vi "Init.vi"(8 "error in (no error)":errorcluster caption="entrée d'erreur (pas d'erreur)", 11 "Class Spectrum_Analyser RS306B en entrée":refnum<class "Class Spectrum_Analyser RS306B.lvclass">) -> (0 "error out":errorcluster caption="sortie d'erreur", 3 "Class Spectrum_Analyser RS306B en sortie":refnum<class "Class Spectrum_Analyser RS306B.lvclass">)   [LabVIEW 2020, in "Library Instrument & Equipement.lvlib" / "Library Spectrum Analyser.lvlib" / "Class Spectrum_Analyser RS306B.lvclass"]
uses:
  Class Spectrum_Analyser RS306B.lvclass
  C:/Users/ngarcin/OneDrive - Altyor/Standard TB/Class/Spectrum Analyser/Class Spectrum Analyser (Default)/Class Spectrum Analyser (Default).lvclass
  Class Spectrum_Analyser RS306B.lvclass/Class Spectrum_Analyser RS306B.ctl
  Library Spectrum Analyser.lvlib
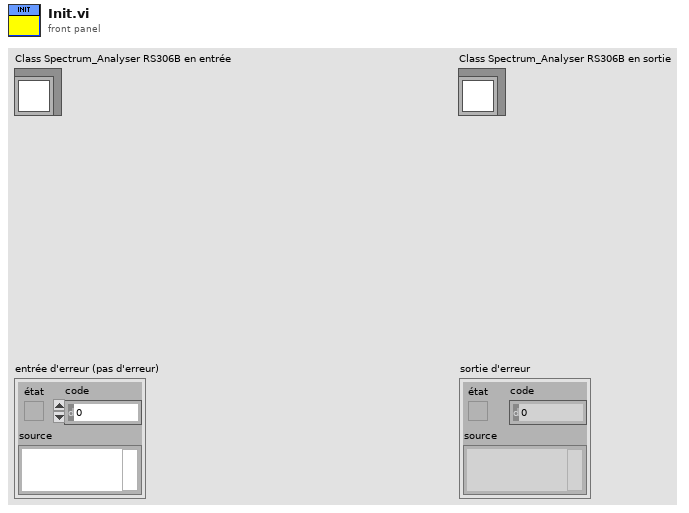
[diagram p1: front panel]
types:
  T1 = enum16{"SEARCH ON", "SEARCH OFF", "SEARCH TRACE", "SEARCH CRITERIA", "SEARCH THRESHOLD", "BEEP ON MATCH ON", "BEEP ON MATCH OFF", "STOP ON MATCH ON", "STOP ON MATCH OFF", "AUTOSAVE ACQ DATA ON MATCH ON", "AUTOSAVE ACQ DATA ON MATCH OFF", "AUTOSAVE TRACE ON MATCH ON", "AUTOSAVE TRACE ON MATCH OFF", "AUTOSAVE PICTURE ON MATCH ON", "AUTOSAVE PICTURE ON MATCH OFF", "SAVE SEARCH MASK TO FILE (SET)", "LOAD SEARCH MASK FROM FILE (SET)", "SEARCH RESULTS (READ)"}
  T2 = enum16{"<  THRESHOLD", "> THRESHOLD", "INSIDE MASK", "OUTSIDE MASK"}
  T3 = enum16{"NORMAL", "AVERAGE", "MAX HOLD", "MIN HOLD", "AVERAGE LOG"}
  T4 = enum16{"TRACE FUNCTION", "TRACE DETECTION", "SELECT TRACE", "TRACE ON", "TRACE OFF", "FREEZE ON", "FREEZE OFF", "AVERAGE COUNT", "CLEAR AVE/MAX/MIN (SET)", "CLEAR TRACES (SET)", "LEFT OPERAND", "RIGHT OPERAND"}
  T5 = enum16{"+PEAK", "-PEAK", "AVERAGE", "SAMPLE", "CISPR AVG", "CISPR PK", "CISPR QPK", "AVERAGE LOG"}
  T6 = enum16{"REFERENCE LEVEL", "RF ATTENUATION", "AUTO ATTENUATION ON", "AUTO ATTENUATION OFF", "PREAMP ON", "PREAMP OFF", "VERTICAL UNITS"}
  T7 = enum16{"CENTER FREQUENCY", "FREQUENCY SPAN", "RESOLUTION BW", "MAX REAL TIME SPAN (SET)", "START FREQUENCY", "STOP FREQUENCY", "FREQ STEP SIZE", "AUTO FREQ STEP ON", "AUTO FREQ STEP OFF", "AUTO RES BW ON", "AUTO RES BW OFF", "FFT WINDOW TYPE", "# POINTS", "RBW PROCESS ON", "RBW PROCESS OFF", "GAIN/BW OPTIMIZATION"}
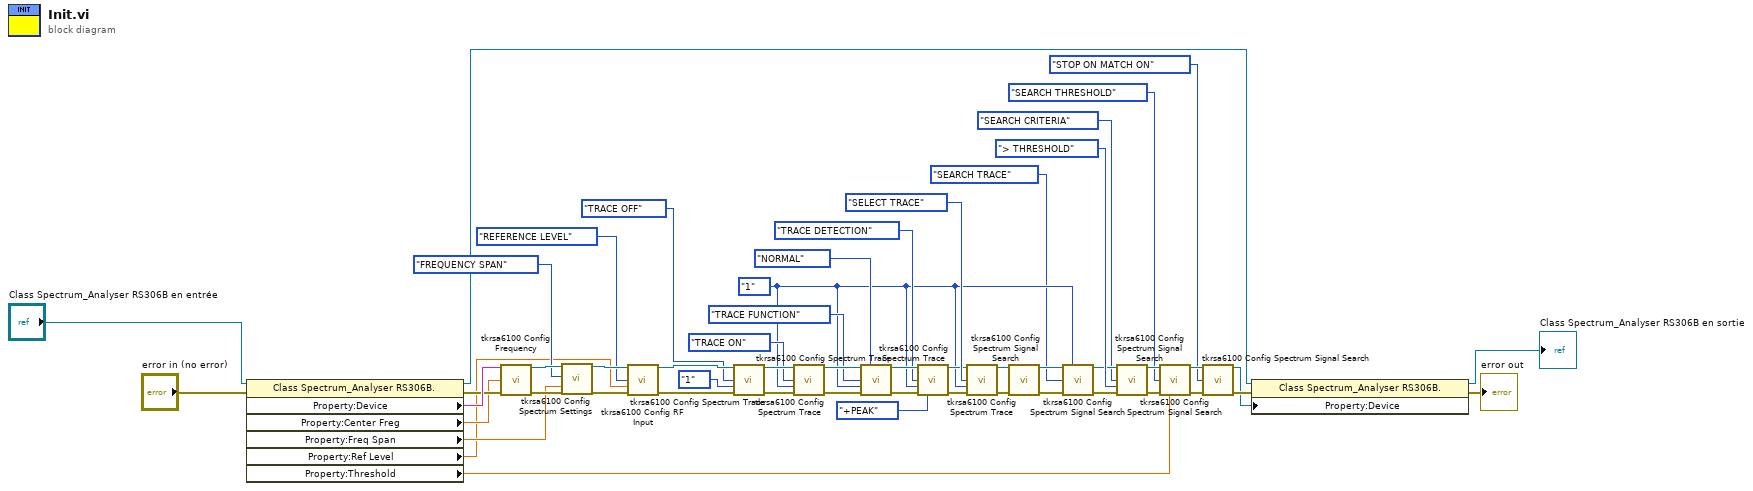
[diagram p0: block diagram]
diagram:
  w27 = enum16{"1", "2", "3", "MATH", "SGRAM"}."1" ("Trace # (1)")
  n1 = property class="Class Spectrum_Analyser RS306B."(reference="Class Spectrum_Analyser RS306B en entrée", error in="error in (no error)") -> (reference out=w8:refnum<class "Class Spectrum_Analyser RS306B.lvclass">, error out=w11:errorcluster, "Property:Device"=w12:string, "Property:Center Freg"=w4:dbl, "Property:Freq Span"=w3:dbl, "Property:Ref Level"=w2:dbl, "Property:Threshold"=w1:dbl)
  n2 = call "tkrsa6100 Config Frequency.vi"("VISA Resource Name"=w12, "Msmt Freq (MHz)\n(1000)"=w4, "error in (no error)"=w11) -> ("dup VISA Resource Name"=w53:refnum<visa-resource-name>, "error out"=w52:errorcluster)  [unwired: 10 in, 1 out]
  n3 = call "tkrsa6100 Config Spectrum Settings.vi"("VISA Resource Name"=w53, "Spectrum Settings\n (CENTER FREQUENCY)"=T7."FREQUENCY SPAN" ("Spectrum Settings\n (CENTER FREQUENCY)"), "Freq Span\n(MHz)(40)"=w3, "error in (no error)"=w52) -> ("dup VISA Resource Name"=w51:refnum<visa-resource-name>, "error out"=w50:errorcluster)  [unwired: 13 in, 1 out]
  n4 = call "tkrsa6100 Config RF Input.vi"("VISA Resource Name"=w51, "Input Settings\n(REFERENCE LEVEL)"=T6."REFERENCE LEVEL" ("Input Settings\n(REFERENCE LEVEL)"), "Ref Level (0)"=w2, "error in (no error)"=w50) -> ("dup VISA Resource Name"=w49:refnum<visa-resource-name>, "error out"=w48:errorcluster)  [unwired: 9 in, 1 out]
  n5 = call "tkrsa6100 Config Spectrum Trace.vi"("VISA Resource Name"=w49, "Trace Setting\n(TRACE FUNCTION)"=T4."TRACE OFF" ("Trace Setting\n(TRACE FUNCTION)"), "Trace # (1)"=enum16{"1", "2", "3", "MATH", "SGRAM"}."1", "error in (no error)"=w48) -> ("dup VISA Resource Name"=w43:refnum<visa-resource-name>, "error out"=w42:errorcluster)  [unwired: 9 in, 1 out]
  n6 = call "tkrsa6100 Config Spectrum Trace.vi"("VISA Resource Name"=w43, "Trace Setting\n(TRACE FUNCTION)"=T4."TRACE ON" ("Trace Setting\n(TRACE FUNCTION)"), "Trace # (1)"=w27, "error in (no error)"=w42) -> ("dup VISA Resource Name"=w38:refnum<visa-resource-name>, "error out"=w39:errorcluster)  [unwired: 9 in, 1 out]
  n7 = call "tkrsa6100 Config Spectrum Trace.vi"("VISA Resource Name"=w38, "Trace Function\n(NORMAL)"=T3."NORMAL" ("Trace Function\n(NORMAL)"), "Trace Setting\n(TRACE FUNCTION)"=T4."TRACE FUNCTION" ("Trace Setting\n(TRACE FUNCTION)"), "Trace # (1)"=w27, "error in (no error)"=w39) -> ("dup VISA Resource Name"=w34:refnum<visa-resource-name>, "error out"=w36:errorcluster)  [unwired: 8 in, 1 out]
  n8 = call "tkrsa6100 Config Spectrum Trace.vi"("VISA Resource Name"=w34, "Trace Setting\n(TRACE FUNCTION)"=T4."TRACE DETECTION" ("Trace Setting\n(TRACE FUNCTION)"), "Trace # (1)"=w27, "error in (no error)"=w36, "Trace Detection\n(+PEAK)"=T5."+PEAK" ("Trace Detection\n(+PEAK)")) -> ("dup VISA Resource Name"=w33:refnum<visa-resource-name>, "error out"=w35:errorcluster)  [unwired: 8 in, 1 out]
  n9 = call "tkrsa6100 Config Spectrum Trace.vi"("VISA Resource Name"=w33, "Trace Setting\n(TRACE FUNCTION)"=T4."SELECT TRACE" ("Trace Setting\n(TRACE FUNCTION)"), "Trace # (1)"=w27, "error in (no error)"=w35) -> ("dup VISA Resource Name"=w29:refnum<visa-resource-name>, "error out"=w28:errorcluster)  [unwired: 9 in, 1 out]
  n10 = call "tkrsa6100 Config Spectrum Signal Search.vi"("VISA Resource Name"=w29, "error in (no error)"=w28) -> ("dup VISA Resource Name"=w26:refnum<visa-resource-name>, "error out"=w25:errorcluster)  [unwired: 10 in, 2 out]
  n11 = call "tkrsa6100 Config Spectrum Signal Search.vi"("VISA Resource Name"=w26, "Trace (1)"=w27, "Search Setting\n(SEARCH ON)"=T1."SEARCH TRACE" ("Search Setting\n(SEARCH ON)"), "error in (no error)"=w25) -> ("dup VISA Resource Name"=w22:refnum<visa-resource-name>, "error out"=w21:errorcluster)  [unwired: 8 in, 2 out]
  n12 = call "tkrsa6100 Config Spectrum Signal Search.vi"("VISA Resource Name"=w22, "Search Setting\n(SEARCH ON)"=T1."SEARCH CRITERIA" ("Search Setting\n(SEARCH ON)"), "Search Criteria\n(< THRESHOLD)"=T2."> THRESHOLD" ("Search Criteria\n(< THRESHOLD)"), "error in (no error)"=w21) -> ("dup VISA Resource Name"=w19:refnum<visa-resource-name>, "error out"=w18:errorcluster)  [unwired: 8 in, 2 out]
  n13 = call "tkrsa6100 Config Spectrum Signal Search.vi"("VISA Resource Name"=w19, "Search Setting\n(SEARCH ON)"=T1."SEARCH THRESHOLD" ("Search Setting\n(SEARCH ON)"), "error in (no error)"=w18, "Threshold (0)"=w1) -> ("dup VISA Resource Name"=w16:refnum<visa-resource-name>, "error out"=w15:errorcluster)  [unwired: 8 in, 2 out]
  n14 = call "tkrsa6100 Config Spectrum Signal Search.vi"("VISA Resource Name"=w16, "Search Setting\n(SEARCH ON)"=T1."STOP ON MATCH ON" ("Search Setting\n(SEARCH ON)"), "error in (no error)"=w15) -> ("dup VISA Resource Name"=w9:refnum<visa-resource-name>, "error out"=w10:errorcluster)  [unwired: 9 in, 2 out]
  n15 = property class="Class Spectrum_Analyser RS306B."(reference=w8, error in=w10, "Property:Device"=w9) -> (reference out=→"Class Spectrum_Analyser RS306B en sortie":refnum<class "Class Spectrum_Analyser RS306B.lvclass">, error out=→"error out":errorcluster)
